vi "PPL Pre-Build CHM Build.vi"(6 "Top Level/Always Included VIs":path[](array[path]), 7 "Main Destination Path":path, 9 "Target Name":string, 10 "Build Specification Name":string, 11 "Project Path":path) -> (0 "error out":errorcluster)   [LabVIEW 2019]
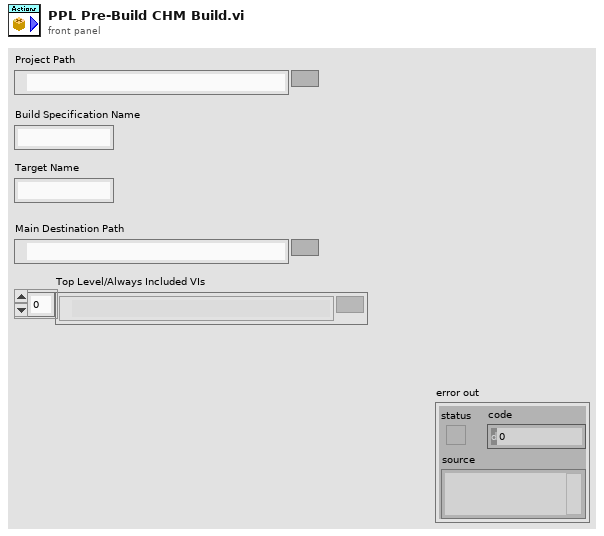
[diagram p1: front panel]
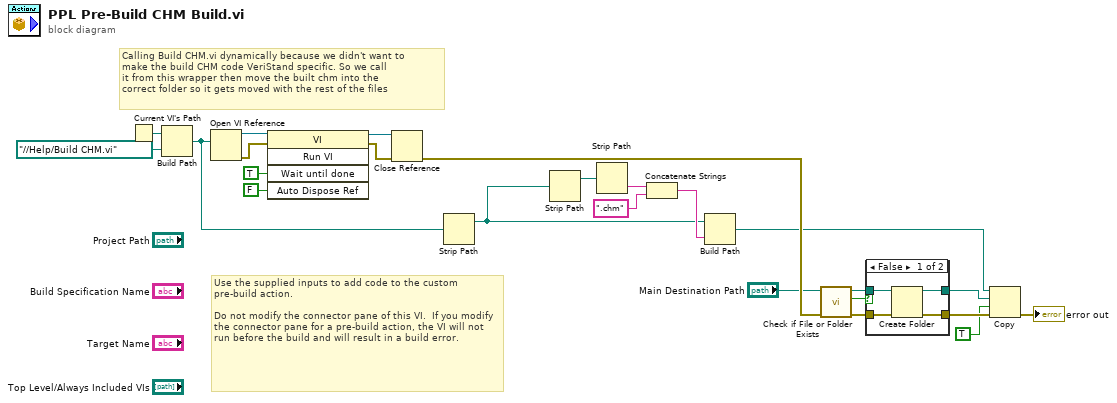
[diagram p0: block diagram]
diagram:
  # "Calling Build CHM.vi dynamically because we didn't want to \nmake the build CHM code VeriStand specific. So we call\nit from this wrapper then move the built chm into the\ncorrect folder so it gets moved with the rest of the files"
  # "Use the supplied inputs to add code to the custom pre-build action.\n\nDo not modify the connector pane of this VI.  If you modify the connector pane for a pre-build action, the VI will not run before the build and will result in a build error."
  n1 = Current VI's Path() -> (path=w24:path)
  n2 = Build Path(base path=w24, name or relative path=path "../../Help/Build CHM.vi") -> (appended path=w16:path)
  n3 = Open VI Reference(vi path=w16) -> (vi reference=w22:refnum<vi>, error out=w21:errorcluster)  [unwired: 5 in]
  n4 = invoke class="VI" method="Run VI"(reference=w22, error in=w21, "Wait until done"=TRUE ("Wait Until Done"), "Auto Dispose Ref"=FALSE ("Auto Dispose Reference")) -> (reference out=w18:refnum<vi>, error out=w17:errorcluster)  [unwired: 1 in, 3 out]
  n5 = Close Reference(reference=w18, error in (no error)=w17) -> (error out=w11:errorcluster)
  n6 = Strip Path(path=w16) -> (stripped path=w2:path)  [unwired: 1 out]
  n7 = Strip Path(path=w2) -> (stripped path=w15:path)  [unwired: 1 out]
  n8 = Strip Path(path=w15) -> (name=w14:string)  [unwired: 1 out]
  n9 = Concatenate Strings(w14, ".chm" ("string")) -> (w12:string)
  n10 = Build Path(base path=w2, name or relative path=w12) -> (appended path=w4:path)
  n11 = call <vilib>:"Check if File or Folder Exists.vi"("error in (no error)"=w11, "path"="Main Destination Path") -> ("error out"=w8:errorcluster, "file or folder exists?"=w10:bool, "dup path"=w9:path)  [unwired: 7 in]
  n12 = case shown="False" w10 {
    tunnel: w9 -> [w27 w30]
    tunnel: w8 -> [w28 w29]
    tunnel: [w26 w30] -> w6
    tunnel: [w25 w29] -> w7
    frame False {
      n13 = Create Folder(path (use dialog)=w27, error in=w28) -> (created path=w26:path, error out=w25:errorcluster)  [unwired: 1 in, 1 out]
    }
    frame True {
    }
  }
  n14 = Copy(8:w7, 9:TRUE ("overwrite (F)"), 10:w6, 11:w4) -> (0:→"error out":errorcluster)  [unwired: 1 in, 2 out]
